vi "CreateVirtualSubFolder.vi"(8 "error in (no error)":errorcluster, 10 "SubFolderArray":string[](array[string]), 11 "ClassLibReference":refnum<vi>) -> (0 "error out":errorcluster, 3 "ActSubFolderRef":refnum<vi>)   [LabVIEW 2014, in "CS++Actor.lvlib" / "CS++Actor.lvclass"]
uses:
  CS++Actor.lvclass
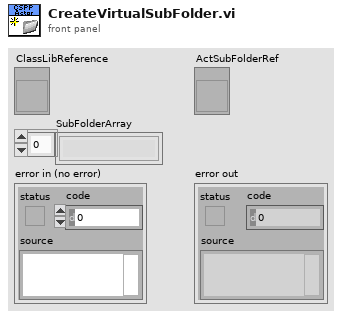
[diagram p1: front panel]
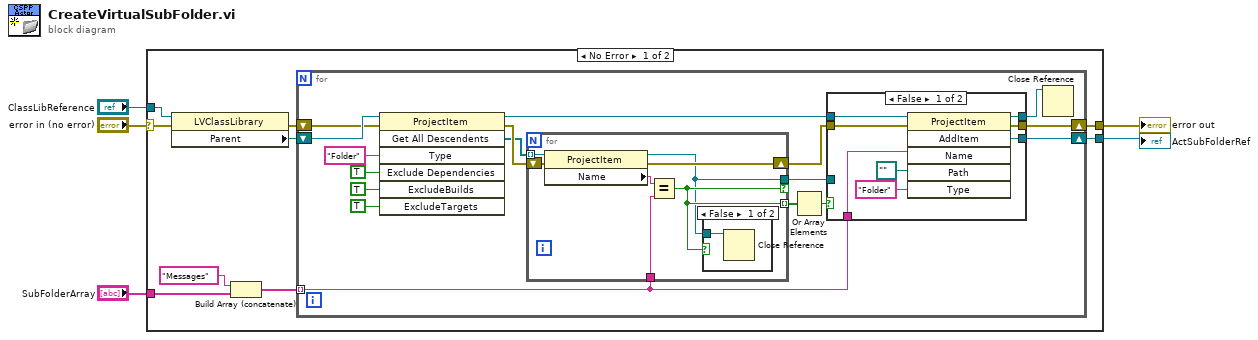
[diagram p0: block diagram]
diagram:
  n1 = case shown="No Error" "error in (no error)" {
    selector: "error in (no error)" -> [w11 w51]
    tunnel: [w10 w51] -> w4
    tunnel: "ClassLibReference" -> [w12 _]
    tunnel: "SubFolderArray" -> [w8 _]
    tunnel: [w6 _] -> w1
    frame No Error {
      n2 = property class="LVClassLibrary"(reference=w12, error in=w11) -> (error out=w13:errorcluster, "Parent"=w14:refnum<vi>)  [unwired: 1 out]
      n3 = Build Array (concatenate)("Messages" ("y"), w8) -> (w7:string[])
      n4 = for {
        shift-right: [w19] -> w10
        shift-left: w13 -> [w29]
        tunnel: w7 -> [w18] mode=indexing
        shift-right: [w17] -> w6
        shift-left: w14 -> [w31]
        n5 = invoke class="ProjectItem" method="Get All Descendents"(reference=w31, error in=w29, "Type"="Folder", "Exclude Dependencies"=TRUE ("ExcludeDependencies"), "ExcludeBuilds"=TRUE, "ExcludeTargets"=TRUE) -> (reference out=w30:refnum<vi>, error out=w24:errorcluster, "All Descendents"=w20:refnum<vi>[])  [unwired: 1 in, 4 out]
        n6 = for {
          tunnel: w20 -> [w49] mode=indexing
          shift-right: [w47] -> w22
          shift-left: w24 -> [w48]
          tunnel: [w43] -> w21 if=w44
          tunnel: [w44] -> w23 mode=indexing
          tunnel: w18 -> [w45]
          n7 = property class="ProjectItem"(reference=w49, error in=w48) -> (reference out=w43:refnum<vi>, error out=w47:errorcluster, "Name"=w46:string)
          n8 = Equal?(x=w46, y=w45) -> (x = y?=w44:bool)
          n9 = case shown="False" w44 {
            tunnel: w43 -> [w50 _]
            frame False {
              n10 = Close Reference(reference=w50) -> ()  [unwired: 1 in, 1 out]
            }
            frame True {
            }
          }
        }
        n11 = Or Array Elements(Boolean array=w23) -> (logical OR=w15:bool)
        n12 = case shown="False" w15 {
          tunnel: [w37 w42] -> w17
          tunnel: [w36 w41] -> w19
          tunnel: w30 -> [w35 w40]
          tunnel: w22 -> [w34 w41]
          tunnel: w21 -> [_ w42]
          tunnel: [w33 w40] -> w16
          tunnel: w18 -> [w32 _]
          frame False {
            n13 = invoke class="ProjectItem" method="AddItem"(reference=w35, error in=w34, "Name"=w32, "Path"=path "", "Type"="Folder") -> (reference out=w33:refnum<vi>, error out=w36:errorcluster, "AddItem"=w37:refnum<vi>)  [unwired: 1 in, 3 out]
          }
          frame True {
          }
        }
        n14 = Close Reference(reference=w16) -> ()  [unwired: 1 in, 1 out]
      }
    }
    frame Error {
    }
  }
  "error out" <- w4
  "ActSubFolderRef" <- w1
